vi "Frame(PICH).vi"() -> ()   [LabVIEW 2013]
panel:
  out "Frame(PICH)":cluster{dbl, i32, bool[], "Type":i32}
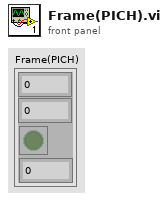
[diagram p1: front panel]
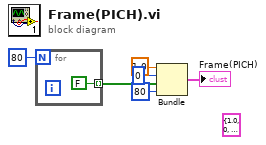
[diagram p0: block diagram]
diagram:
  (unwired) cluster{dbl, i32, bool[], "Type":i32} {1.0, 0, [FALSE, FALSE, FALSE, FALSE, FALSE, FALSE, FALSE, FALSE, FALSE, FALSE, FALSE, FALSE, FALSE, FALSE, FALSE, FALSE, FALSE, FALSE, FALSE, FALSE, FALSE, FALSE, FALSE, FALSE, FALSE, FALSE, FALSE, FALSE, FALSE, FALSE, FALSE, FALSE, FALSE, FALSE, FALSE, FALSE, FALSE, FALSE, FALSE, FALSE, FALSE, FALSE, FALSE, FALSE, FALSE, FALSE, FALSE, FALSE, FALSE, FALSE, FALSE, FALSE, FALSE, FALSE, FALSE, FALSE, FALSE, FALSE, FALSE, FALSE, FALSE, FALSE, FALSE, FALSE, FALSE, FALSE, FALSE, FALSE, FALSE, FALSE, FALSE, FALSE, FALSE, FALSE, FALSE, FALSE, FALSE, FALSE, FALSE, FALSE], "Type"=80} ("Frame(PICH) 2")
  n1 = for {
    N: 80 -> [_]
    tunnel: [FALSE] -> w5 mode=indexing
  }
  n2 = Bundle(1.0, 0, w5, 80) -> (→"Frame(PICH)":cluster{dbl, i32, bool[], i32})  [unwired: 1 in]
